vi "Delete Items from Targets.vi"(8 "error in (no error)":errorcluster, 9 "Items":T1[](array[typedef]), 10 "Targets in":string[](array[string]), 11 "Project Sync Tools in":refnum<class "Project Sync Tools.lvclass">) -> (0 "error out":errorcluster, 1 "Items out":T1[](array[typedef]), 2 "Targets out":string[](array[string]), 3 "Project Sync Tools out":refnum<class "Project Sync Tools.lvclass">)   [LabVIEW 2019, in "Project Sync Tools.lvclass"]
uses:
  Project Sync Tools.lvclass
  TypeDefs/Item Settings.ctl
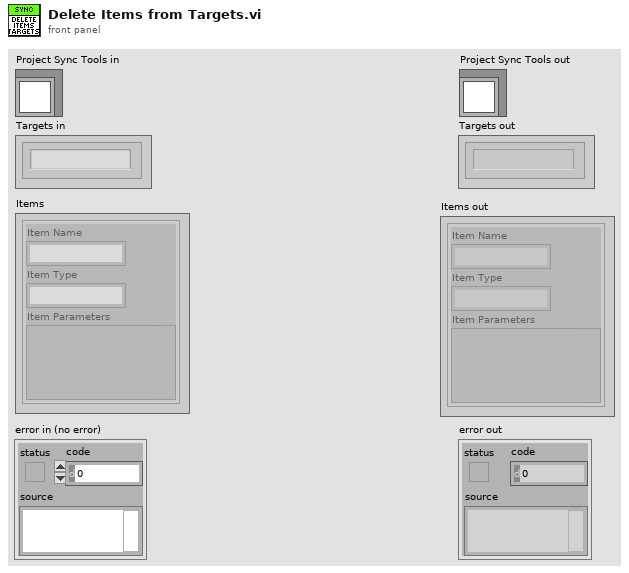
[diagram p1: front panel]
types:
  T1 = typedef "Project Sync Tools.lvclass/Item Settings.ctl" = cluster{"Item Name":string, "Item Type":string, "Item Parameters":variant}
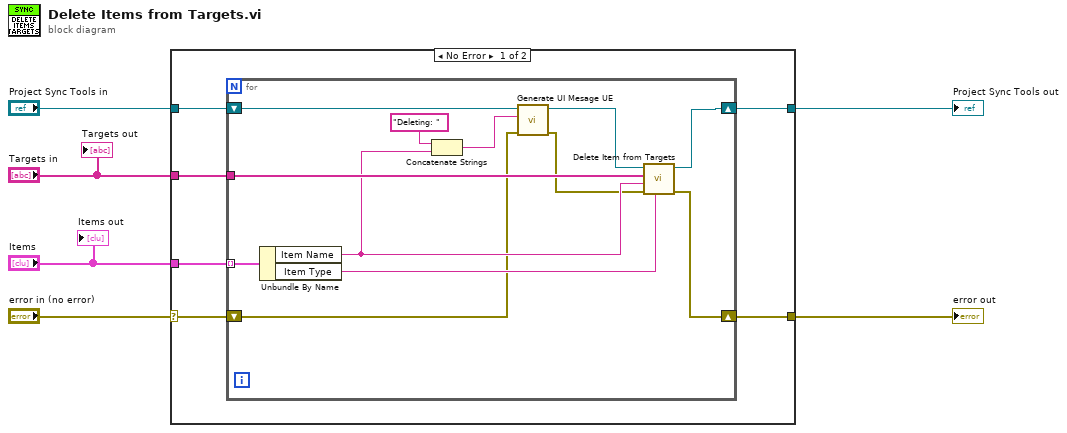
[diagram p0: block diagram]
diagram:
  n1 = case shown="No Error" "error in (no error)" {
    selector: "error in (no error)" -> [w9 w26]
    tunnel: [w7 w26] -> w5
    tunnel: [w8 w25] -> w3
    tunnel: "Project Sync Tools in" -> [w12 w25]
    tunnel: "Targets in" -> [w10 _]
    tunnel: "Items" -> [w11 _]
    frame No Error {
      n2 = for {
        tunnel: w11 -> [w23] mode=indexing
        tunnel: w10 -> [w24]
        shift-right: [w20] -> w8
        shift-left: w12 -> [w17]
        shift-right: [w21] -> w7
        shift-left: w9 -> [w14]
        n3 = Unbundle By Name(w23) -> ("Item Name"=w18:string, "Item Type"=w22:string)
        n4 = Concatenate Strings("Deleting: " ("string"), w18) -> (w15:string)
        n5 = call "Generate UI Mesage UE.vi"("error in (no error)"=w14, "UI Message"=w15, "Project Sync Tools in"=w17) -> ("error out"=w13:errorcluster, "Project Sync Tools out"=w16:refnum<class "Project Sync Tools.lvclass">)  [unwired: 7 in]
        n6 = call "Delete Item from Targets.vi"("Type"=w22, "error in (no error)"=w13, "Item Name"=w18, "Target Names in"=w24, "Project Sync Tools in"=w16) -> ("error out"=w21:errorcluster, "Project Sync Tools out"=w20:refnum<class "Project Sync Tools.lvclass">)  [unwired: 4 in, 1 out]
      }
    }
    frame Error {
    }
  }
  "error out" <- w5
  "Project Sync Tools out" <- w3
  "Targets out" <- "Targets in"
  "Items out" <- "Items"
